vi "user32_CascadeWindows.vi"(0 "hWndParent":u32, 1 "wHow":u32(ring) items=["VERTICAL", "HORIZONTAL", ""], 5 "lpRect":T1, 7 "cKids":u32, 9 "lpKids":u32, 11 "错误输入（无错误）":errorcluster) -> (4 "dup hWndParent":u32, 6 "ArrangedWindowNum":i32, 15 "错误输出":errorcluster)   [LabVIEW 2011]
doc: "以层叠方式排列窗口。"
uses:
  user32.dll
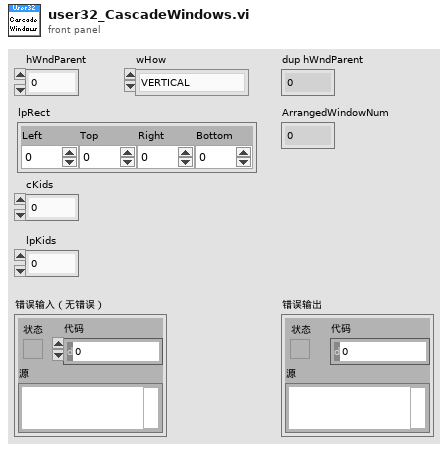
[diagram p1: front panel]
types:
  T1 = cluster{"Left":i32, "Top":i32, "Right":i32, "Bottom":i32}
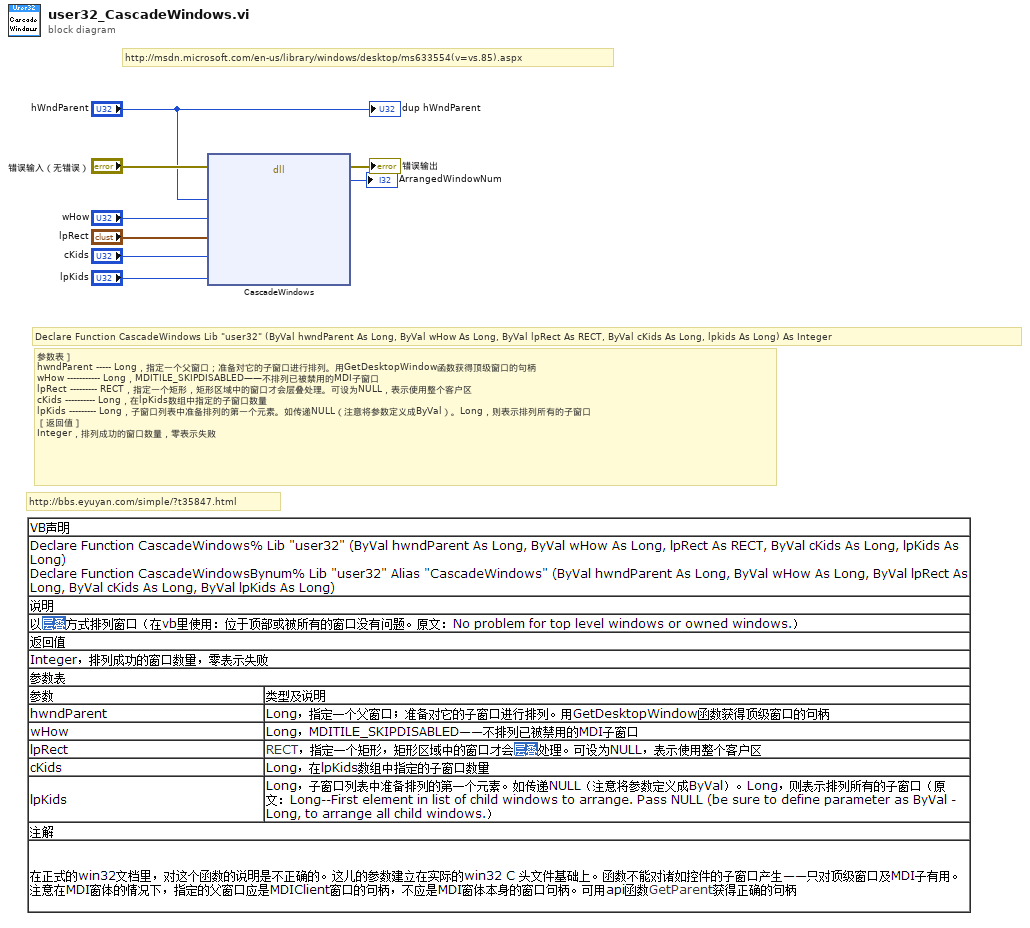
[diagram p0: block diagram]
diagram:
  # "http://msdn.microsoft.com/en-us/library/windows/desktop/ms633554(v=vs.85).aspx"
  # "http://bbs.eyuyan.com/simple/?t35847.html"
  # "参数表］\nhwndParent ----- Long，指定一个父窗口；准备对它的子窗口进行排列。用GetDesktopWindow函数获得顶级窗口的句柄\nwHow ----------- Long，MDITILE_SKIPDISABLED——不排列已被禁用的MDI子窗口\nlpRect --------- RECT，指定一个矩形，矩形区域中的窗口才会层叠处理。可设为NULL，表示使用整个客户区\ncKids ---------- Long，在lpKids数组中指定的子窗口数量\nlpKids --------- Long，子窗口列表中准备排列的第一个元素。如传递NULL（注意将参数定义成ByVal）。Long，则表示排列所有的子窗口\n［返回值］\nInteger，排列成功的窗口数量，零表示失败"
  # "Declare Function CascadeWindows Lib \"user32\" (ByVal hwndParent As Long, ByVal wHow As Long, ByVal lpRect As RECT, ByVal cKids As Long, lpkids As Long) As Integer"
  n1 = dll-call lib="user32.dll" fn="CascadeWindows"(error in="错误输入（无错误）", "hWndParent"="hWndParent", "wHow"="wHow", "lpRect"="lpRect", "cKids"="cKids", "lpKids"="lpKids") -> (error out=→"错误输出":errorcluster, "ArrangedWNum"=→"ArrangedWindowNum":i32)  [unwired: 7 in, 1 out]
  "dup hWndParent" <- "hWndParent"
